vi "DDS Motor Test.vi"() -> ()   [LabVIEW 2021]
uses:
  <vilib>/RTI DDS Toolkit/Types/RTI DDS Advanced Writer Configuration.ctl
  <vilib>/Platform/TimedLoop/XDataNode/timing_clust.ctl
  <vilib>/Platform/TimedLoop/XDataNode/nitl_modes.ctl
  <vilib>/Platform/TimedLoop/XDataNode/wakeup.ctl
  <vilib>/RTI DDS Toolkit/VIs/AdvancedCreateWriter_NumI32.vi
  <vilib>/RTI DDS Toolkit/VIs/Write_NumI32.vi
  <vilib>/Platform/TimedLoop/XDataNode/XDataNode.xnode
  <vilib>/RTI DDS Toolkit/Library/LVDDS_library.lvlib
  <vilib>/Platform/TimedLoop/XDataNode/XDNodeRunTimeDep.lvlib
panel:
  in  "Advanced Writer Configuration":T1={"typeName"="std_msgs::msg::dds_::Int32_", "keyName"="", "domainParticipantQoSProfile"="", "dataWriterQoSProfile"="", "forceArrayMapping?"=FALSE, "forceUnboundedString?"=FALSE}
  in  "stop":bool
  # "DDS Communication"
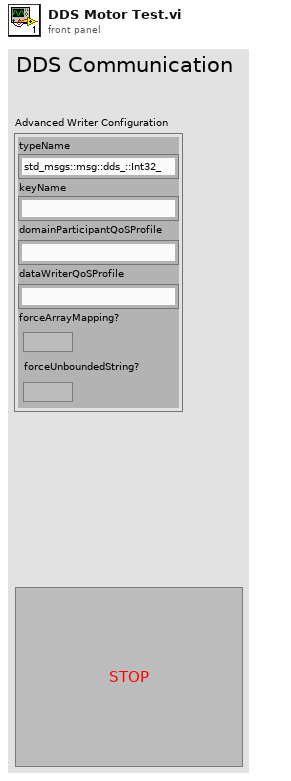
[diagram p1: front panel]
types:
  T1 = typedef "LVDDS_library.lvlib/RTI DDS Advanced Writer Configuration.ctl" = cluster{"typeName":string, "keyName":string, "domainParticipantQoSProfile":string, "dataWriterQoSProfile":string, "forceArrayMapping?":bool, "forceUnboundedString?":bool}
  T2 = typedef "XDNodeRunTimeDep.lvlib/timing_clust.ctl" = cluster{"Expected End [f-1]":u64, "Actual End [f-1]":u64, "Finished Late? [f-1]":bool, "Expected End [i-1]":u64, "Actual End [i-1]":u64, "Finished Late? [i-1]":bool, "Expected Start [i]":u64, "Actual Start [i]":u64, "Expected Start [f]":u64, "Actual Start [f]":u64, "Source Name":string, "Structure Name":string, "Period":i64, "Deadline":i64, "Offset":i64, "Start":i64, "Priority":i32, "Timeout":i32, "Mode":T3, "Wakeup Reason":T4, "Error":errorcluster, "Source Type":string, "Secondary Source Type":string, "Global End Time":u64, "Global Start Time":u64, "Frame Duration":u64, "Iteration Duration":u64, "Assigned CPU":i32, "I/O Scan Engine Mode":u32}
  T3 = typedef "XDNodeRunTimeDep.lvlib/nitl_modes.ctl" = enum32{"No Change", "Process missed periods, maintain original phase", "Discard missed periods, maintain original phase", "Process missed periods, ignore original phase", "Discard missed periods, ignore original phase"}
  T4 = typedef "XDNodeRunTimeDep.lvlib/wakeup.ctl" = enum32{"Normal", "Aborted", "Asynchronous wakeup", "Timing source error", "Timed loop error", "Timeout"}
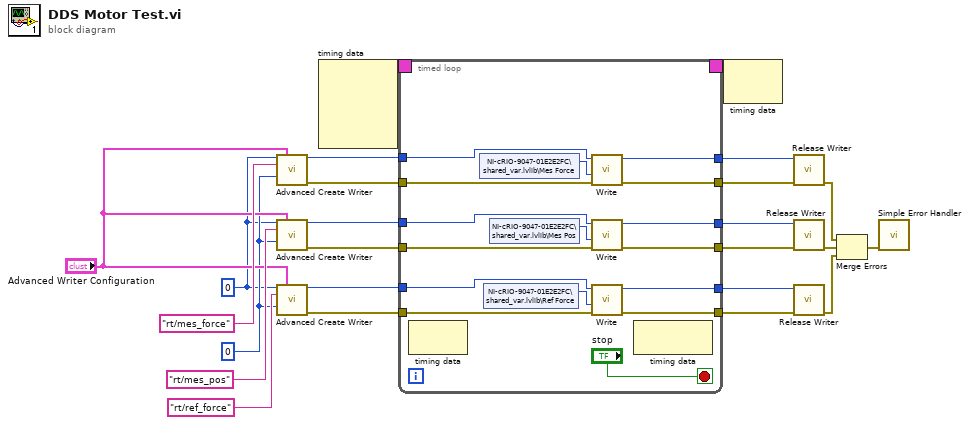
[diagram p0: block diagram]
diagram:
  w3 = 0 ("Data Type")
  w2 = u32 0 ("Domain Id")
  n1 = call-poly <vilib>:"Advanced Create Writer.vi"("Domain Id"=w2, "Advanced Writer Configuration"="Advanced Writer Configuration", "Topic Name"="rt/mes_force", "Data Type"=w3) -> ("DDS Object Ref"=w16:u64, "error out"=w15:errorcluster)  [unwired: 10 in]
  n2 = call-poly <vilib>:"Advanced Create Writer.vi"("Domain Id"=w2, "Advanced Writer Configuration"="Advanced Writer Configuration", "Topic Name"="rt/mes_pos", "Data Type"=w3) -> ("DDS Object Ref"=w23:u64, "error out"=w22:errorcluster)  [unwired: 10 in]
  n3 = call-poly <vilib>:"Advanced Create Writer.vi"("Domain Id"=w2, "Advanced Writer Configuration"="Advanced Writer Configuration", "Topic Name"="rt/ref_force", "Data Type"=w3) -> ("DDS Object Ref"=w7:u64, "error out"=w8:errorcluster)  [unwired: 10 in]
  n4 = node-c288() -> (w20:T2)  [unwired: 4 in]
  n5 = timed-loop {
    timing: w20 -> [_]
    timing-out: [_] -> w19
    tunnel: w23 -> [w40]
    tunnel: w22 -> [w39]
    tunnel: [w38] -> w18
    tunnel: [w37] -> w17
    tunnel: w16 -> [w32]
    tunnel: w15 -> [w33]
    tunnel: [w36] -> w14
    tunnel: [w35] -> w13
    tunnel: w8 -> [w31]
    tunnel: w7 -> [w30]
    tunnel: [w29] -> w6
    tunnel: [w28] -> w5
    stop <- "stop" stop-if-true
    n6 = node-c288() -> ()  [unwired: 1 in, 1 out]
    n7 = shared-variable "NI-cRIO-9047-01E2E2FC\\shared_var.lvlib\\Mes Force"() -> (w25:i32)  [unwired: 1 in, 1 out]
    n8 = shared-variable "NI-cRIO-9047-01E2E2FC\\shared_var.lvlib\\Ref Force"() -> (w27:i32)  [unwired: 1 in, 1 out]
    n9 = shared-variable "NI-cRIO-9047-01E2E2FC\\shared_var.lvlib\\Mes Pos"() -> (w26:i32)  [unwired: 1 in, 1 out]
    n10 = call-poly <vilib>:"Write.vi"("error in (no error)"=w33, "Data"=w25, "DDS Object Ref in"=w32) -> ("error out"=w35:errorcluster, "DDS Object Ref out"=w36:u64)  [unwired: 7 in]
    n11 = call-poly <vilib>:"Write.vi"("error in (no error)"=w39, "Data"=w26, "DDS Object Ref in"=w40) -> ("error out"=w37:errorcluster, "DDS Object Ref out"=w38:u64)  [unwired: 7 in]
    n12 = call-poly <vilib>:"Write.vi"("error in (no error)"=w31, "Data"=w27, "DDS Object Ref in"=w30) -> ("error out"=w28:errorcluster, "DDS Object Ref out"=w29:u64)  [unwired: 7 in]
    n13 = node-c288() -> ()  [unwired: 1 in, 1 out]
  }
  n14 = node-c288(w19) -> ()  [unwired: 1 out]
  n15 = call <vilib>:"Release Writer.vi"("error in (no error)"=w13, "DDS Object Ref"=w14) -> ("error out"=w10:errorcluster)  [unwired: 9 in]
  n16 = call <vilib>:"Release Writer.vi"("error in (no error)"=w17, "DDS Object Ref"=w18) -> ("error out"=w12:errorcluster)  [unwired: 9 in]
  n17 = call <vilib>:"Release Writer.vi"("error in (no error)"=w5, "DDS Object Ref"=w6) -> ("error out"=w1:errorcluster)  [unwired: 9 in]
  n18 = Merge Errors(w10, w12, w1) -> (w11:errorcluster)
  n19 = call <vilib>:"Simple Error Handler.vi"("error in (no error)"=w11) -> ()  [unwired: 4 in, 5 out]
